vi "cRIO FPGA ReadWrite EEPROM.vi"(1 "Command":enum8{"Read", "Write"}(ring), 2 "Address":u16, 3 "Data To Write":u8, 4 "Timeout (ms)":u8) -> (14 "Timeout":bool, 16 "Data Read":u8 format="%.0x")   [LabVIEW 2015]
uses:
  <vilib>/eio/EIONode/EIONode.xnode
  Instance           1 34Saved   cRIO FPGA - control eeprom .vi
  Instance           4 34Saved   cRIO FPGA - control eeprom .vi
  Instance           5 34Saved   cRIO FPGA - control eeprom .vi
  <vilib>/rvi/eio/common/nirviEmuTemplateMethod_errors.vi
panel:
  in  "Wakeup wait (ms)":u32=200
  in  "Stop":bool
  in  "Execute":bool
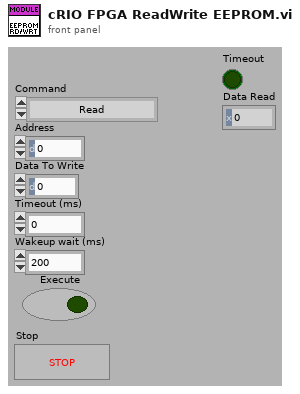
[diagram p1: front panel]
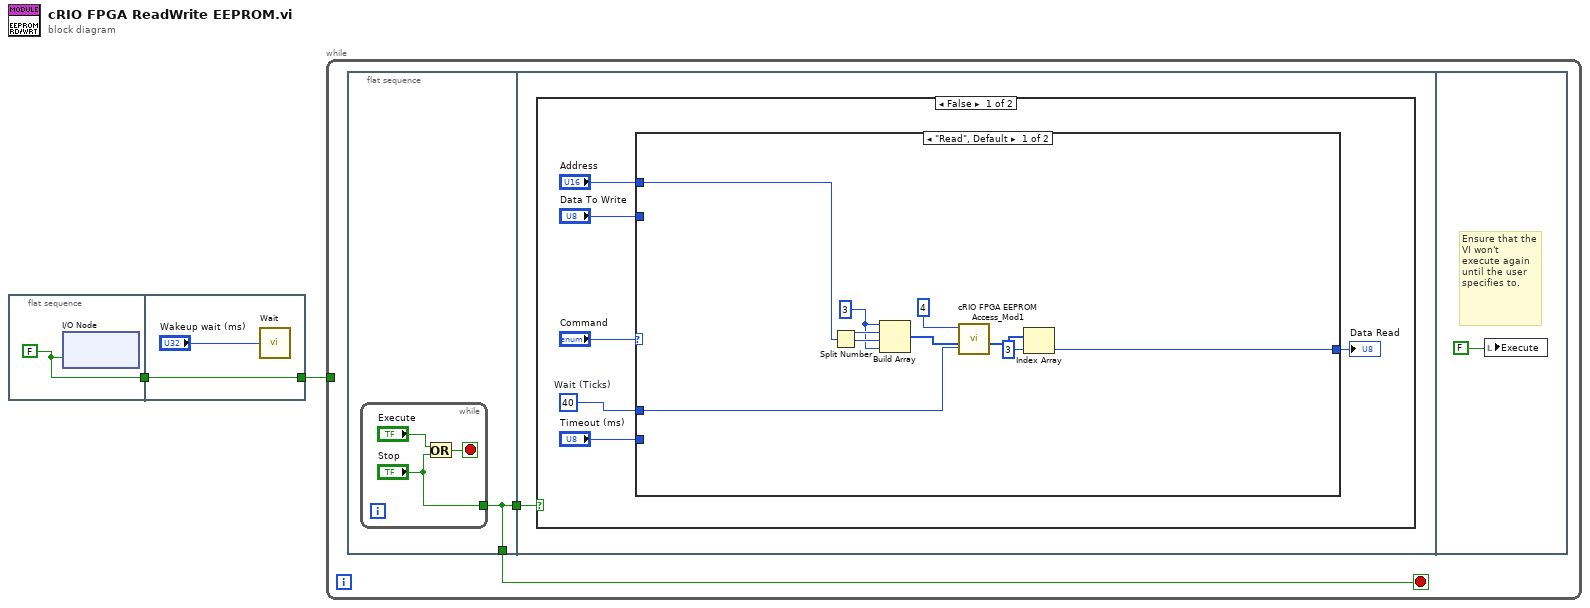
[diagram p0: block diagram]
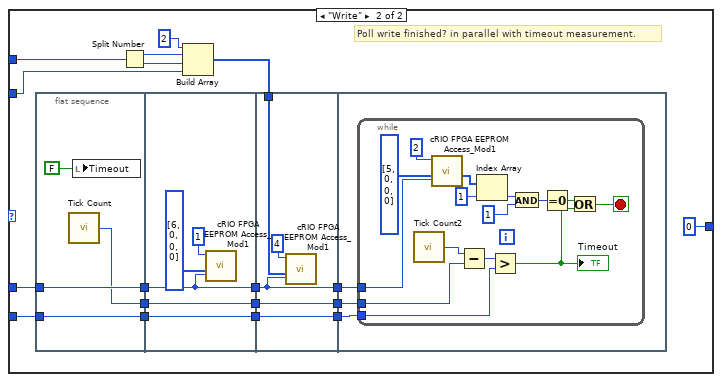
[diagram p2: hidden frame]
diagram:
  n1 = flat-sequence {
    tunnel: [w3] -> w2
    tunnel: [w4] -> w1
    tunnel: w2 -> [w4]
    frame #0 {
      w3 = FALSE ("Digital Out")
      n2 = xnode "I/O Node"("Sleep"=w3) -> ()  [unwired: 1 in, 1 out]
    }
    frame #1 {
      n3 = call "Wait"("Count(mSec)"="Wakeup wait (ms)") -> ()  [unwired: 1 out]
    }
  }
  n4 = while {
    tunnel: w1 -> [_]
    stop <- w6 stop-if-true
    n5 = flat-sequence {
      tunnel: [w8] -> w7
      tunnel: [w8] -> w6
      tunnel: w7 -> [w12]
      frame #0 {
        n6 = while {
          tunnel: ["Stop"] -> w8
          stop <- w11 stop-if-true
          n7 = Or(x="Execute", y="Stop") -> (x .or. y?=w11:bool)
        }
      }
      frame #1 {
        n8 = case shown="False" w12 {
          frame False {
            w15 = u8 40  # Wait (Ticks)
            n9 = case shown="\"Read\", Default" "Command" {
              tunnel: "Data To Write" -> [_ w40]
              tunnel: "Address" -> [w26 w46]
              tunnel: [w28 u8 0] -> w18
              tunnel: w15 -> [w27 w36]
              tunnel: "Timeout (ms)" -> [_ w29]
              frame "Read", Default {
                w23 = u8 3
                n10 = Split Number(x=w26) -> (hi(x)=w25:u8, lo(x)=w24:u8)
                n11 = Build Array(w23, w25, w24, w23) -> (w22:u8[])
                n12 = call "cRIO FPGA EEPROM Access_Mod1.vi"("Wait (Ticks)"=w27, "Data in"=w22, "bytes"=u8 4) -> ("Data out"=w20:u8[])  [unwired: 8 in]
                n13 = Index Array(array=w20, index=3) -> (element=w28:u8)
              }
              frame "Write" {
                # "Poll write finished? in parallel with timeout measurement."
                n14 = flat-sequence {
                  tunnel: w36 -> [w50]
                  tunnel: [w50] -> w37
                  tunnel: [w49] -> w35
                  tunnel: [w48] -> w30
                  tunnel: w29 -> [w48]
                  tunnel: [w53] -> w39
                  tunnel: w37 -> [w53]
                  tunnel: w35 -> [w52]
                  tunnel: [w52] -> w33
                  tunnel: [w51] -> w31
                  tunnel: w30 -> [w51]
                  tunnel: w43 -> [w59]
                  tunnel: w39 -> [w58]
                  tunnel: [w58] -> w38
                  tunnel: [w57] -> w34
                  tunnel: w33 -> [w57]
                  tunnel: [w56] -> w32
                  tunnel: w31 -> [w56]
                  tunnel: w38 -> [w63]
                  tunnel: w34 -> [w62]
                  tunnel: w32 -> [w61]
                  frame #0 {
                    n15 = call "Tick Count"() -> ("Tick Count(mSec)"=w49:u8)
                    n16 = local write "Timeout"(FALSE ("Timeout")) -> ()
                  }
                  frame #1 {
                    n17 = call "cRIO FPGA EEPROM Access_Mod1.vi"("Wait (Ticks)"=w53, "Data in"=u8[] [6, 0, 0, 0] ("in"), "bytes"=u8 1) -> ()  [unwired: 8 in, 1 out]
                  }
                  frame #2 {
                    n18 = call "cRIO FPGA EEPROM Access_Mod1.vi"("Wait (Ticks)"=w58, "Data in"=w59, "bytes"=u8 4) -> ()  [unwired: 8 in, 1 out]
                  }
                  frame #3 {
                    n19 = while {
                      tunnel: w63 -> [w71]
                      tunnel: w62 -> [w69]
                      tunnel: w61 -> [w64]
                      stop <- w66 stop-if-true
                      n20 = call "Tick Count2"() -> ("Tick Count(mSec)"=w70:u8)
                      n21 = call "cRIO FPGA EEPROM Access_Mod1.vi"("Wait (Ticks)"=w71, "Data in"=u8[] [5, 0, 0, 0] ("in"), "bytes"=u8 2) -> ("Data out"=w76:u8[])  [unwired: 8 in]
                      n22 = Subtract(x=w70, y=w69) -> (x-y=w68:u8)
                      n23 = Index Array(array=w76, index=1) -> (element=w74:u8)
                      n24 = Greater?(x=w68, y=w64) -> (0:w65:bool)
                      "Timeout" <- w65
                      n25 = And(x=w74, y=u8 1) -> (x .and. y?=w72:u8)
                      n26 = Equal To 0?(x=w72) -> (x = 0?=w67:bool)
                      n27 = Or(x=w67, y=w65) -> (x .or. y?=w66:bool)
                    }
                  }
                }
                n28 = Split Number(x=w46) -> (hi(x)=w45:u8, lo(x)=w41:u8)
                n29 = Build Array(u8 2 ("element"), w45, w41, w40) -> (w43:u8[])
              }
            }
            "Data Read" <- w18
          }
          frame True {
          }
        }
      }
      frame #2 {
        # "Ensure that the VI won't execute again until the user specifies to."
        n30 = local write "Execute"(FALSE) -> ()
      }
    }
  }
